vi "get Message Event.vi"(8 "error in (no error)":errorcluster, 11 "Messenger - Actor in":refnum<class "Messenger.lvclass">) -> (0 "error out":errorcluster, 2 "Message Event":refnum<user-event>, 3 "Messenger - Actor out":refnum<class "Messenger.lvclass">)   [LabVIEW 2015, in "Messenger.lvclass"]
uses:
  Messenger.lvclass
  Message/Message.lvclass
  Messenger.lvclass/Messenger.ctl
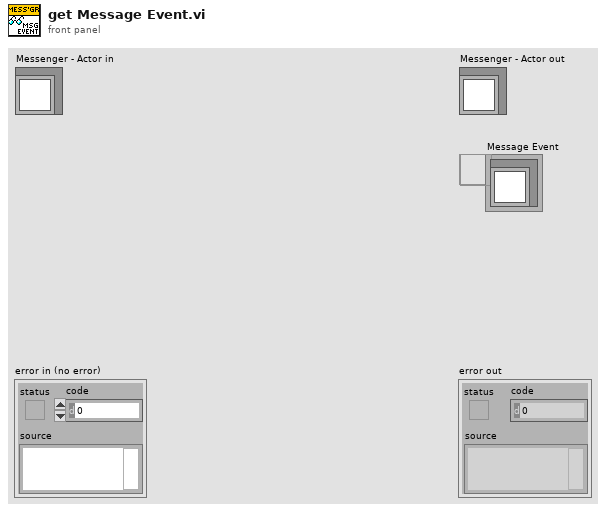
[diagram p1: front panel]
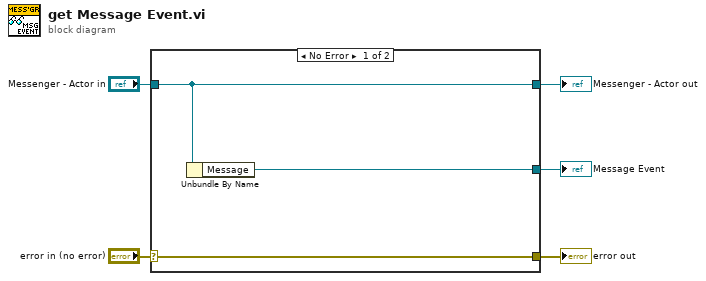
[diagram p0: block diagram]
diagram:
  n1 = case shown="No Error" "error in (no error)" {
    selector: "error in (no error)" -> [w8 w9]
    tunnel: [w8 w9] -> w4
    tunnel: [w7 w10] -> w2
    tunnel: "Messenger - Actor in" -> [w7 w10]
    tunnel: [w6 _] -> w1
    frame No Error {
      n2 = Unbundle By Name(w7) -> ("Message"=w6:refnum<user-event>)
    }
    frame Error {
    }
  }
  "error out" <- w4
  "Messenger - Actor out" <- w2
  "Message Event" <- w1
